vi "SumAroundPeak_10HzFFT.vi"(10 "spectrum in":dbl[](array[numeric])) -> (1 "SumOfPeak":dbl, 2 "MaxValue":dbl, 3 "MaxIndex":i32)   [LabVIEW 2018]
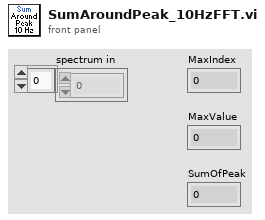
[diagram p1: front panel]
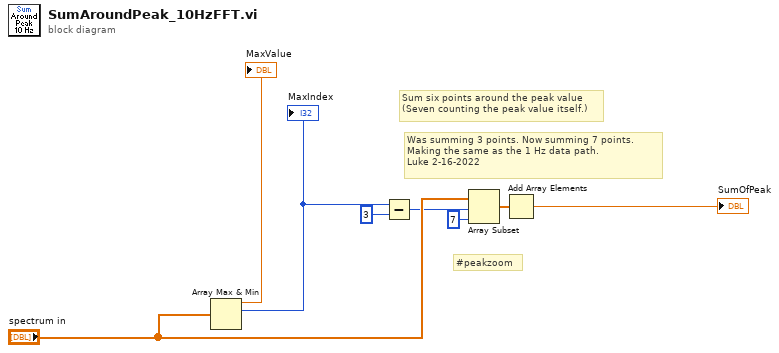
[diagram p0: block diagram]
diagram:
  # "Was summing 3 points. Now summing 7 points.\nMaking the same as the 1 Hz data path.\nLuke 2-16-2022"
  # "#peakzoom"
  # "Sum six points around the peak value\n(Seven counting the peak value itself.)"
  n1 = Array Max & Min(array="spectrum in") -> (max value=→"MaxValue":dbl, max index (indices)=w2:i32)  [unwired: 2 out]
  "MaxIndex" <- w2
  n2 = Subtract(x=w2, y=3) -> (x-y=w4:i32)
  n3 = Array Subset(array="spectrum in", index=w4, length=7) -> (w7:dbl[])
  n4 = Add Array Elements(numeric array=w7) -> (sum=→"SumOfPeak":dbl)
